vi "00_action_FISH02.vi"(11 "Line":string) -> (0 "Command Error":errorcluster, 1 "Execution Return":errorcluster, 2 "Return":string, 3 "full log":string)   [LabVIEW 2019]
uses:
  device/device_global.vi
  device/KQZ1-MP.llb/KQZ1.lvclass
  device/RHEODYNE7970_ADN.llb/RD7970ADN.lvclass
  device/VICI EMHCA.llb/VICI EMHCA_10PORTS.lvclass
  device/MSP1C2.llb/MSP1C2.lvclass
  device/CAVRO_XC.llb/XC3P.lvclass
  device/SC300.llb/SC300.lvclass
  device/SV_LG16ch.llb/SV_LG16ch.lvclass
  device/TETECH_TC720.llb/TC720.lvclass
panel:
  out "Boolean":bool
  out "#number":i32
  out "#class":string
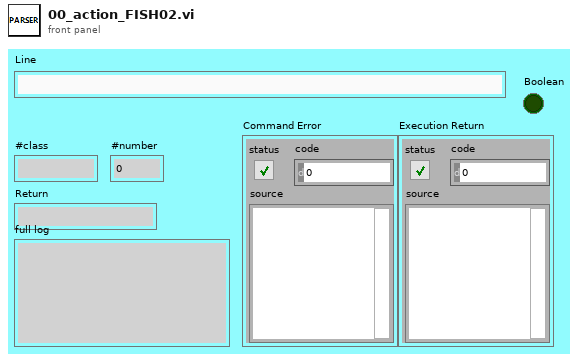
[diagram p1: front panel]
types:
  T1 = enum16{"open", "replace", "create", "open or create", "replace or create", "replace or create with confirmation"}
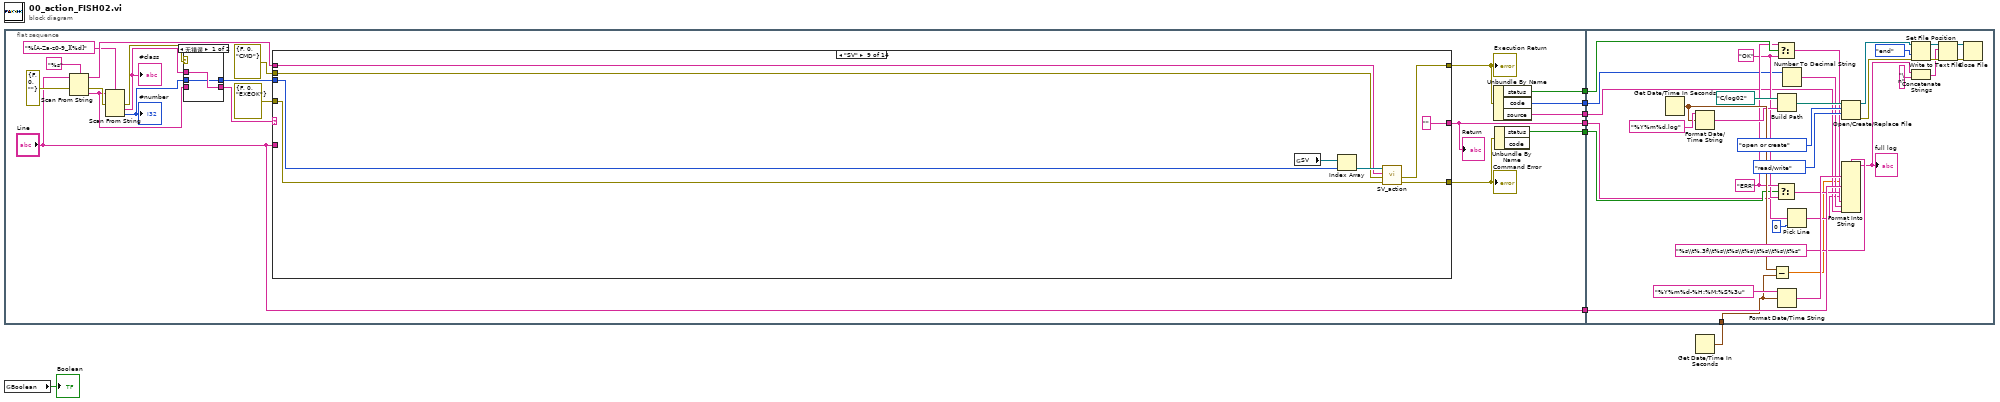
[diagram p0: block diagram]
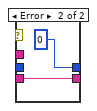
[diagram p2: hidden frame]
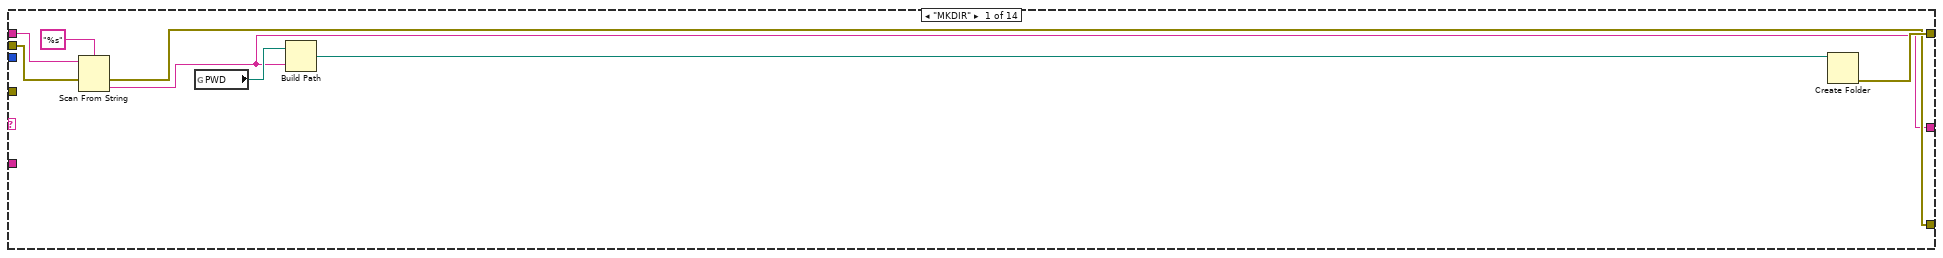
[diagram p3: hidden frame]
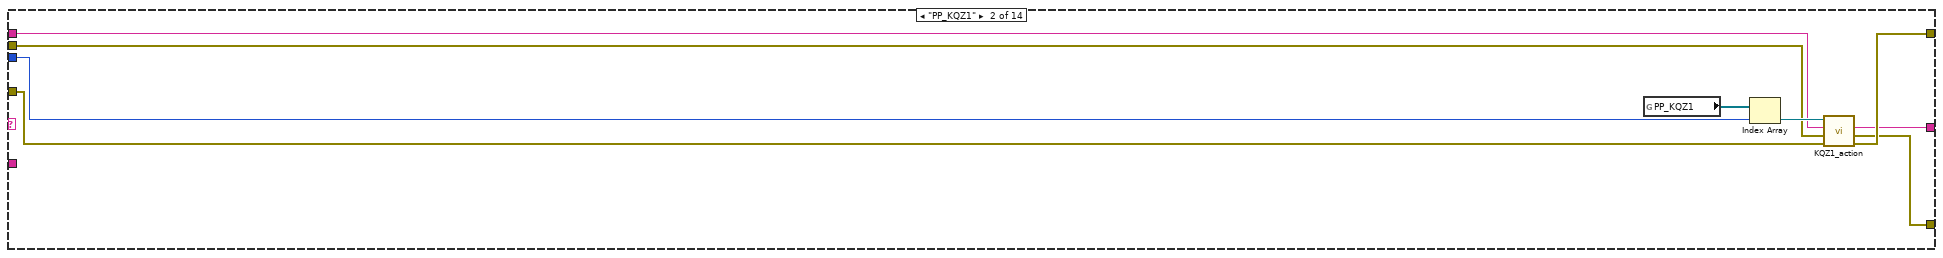
[diagram p4: hidden frame]
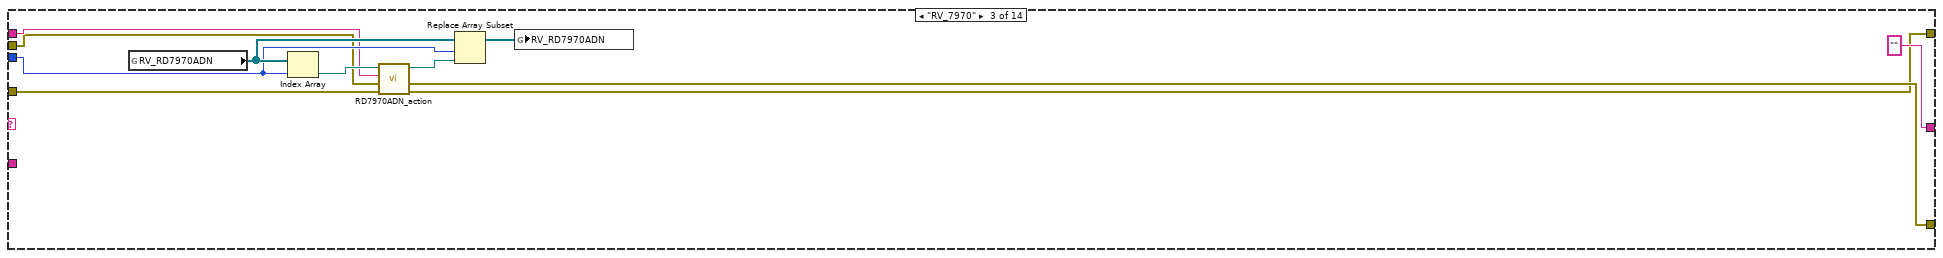
[diagram p5: hidden frame]
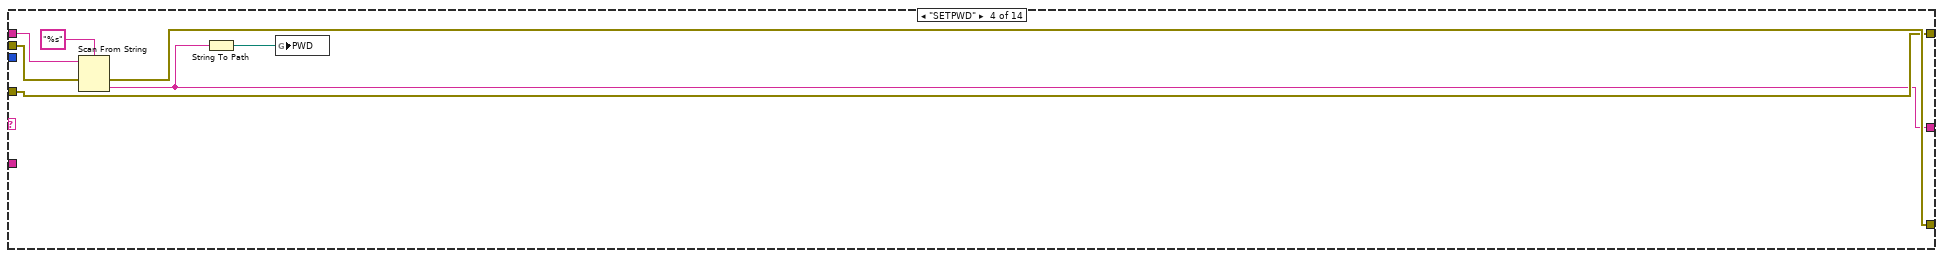
[diagram p6: hidden frame]
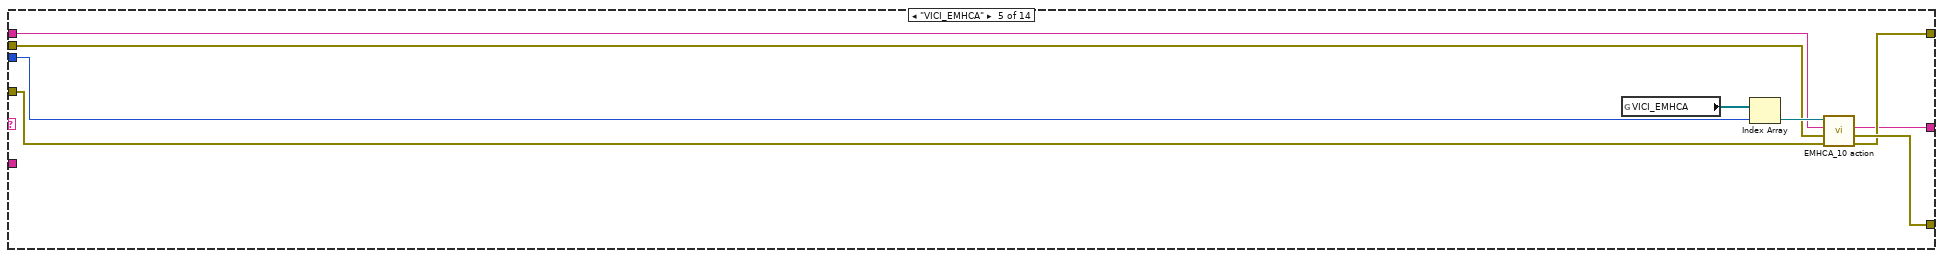
[diagram p7: hidden frame]
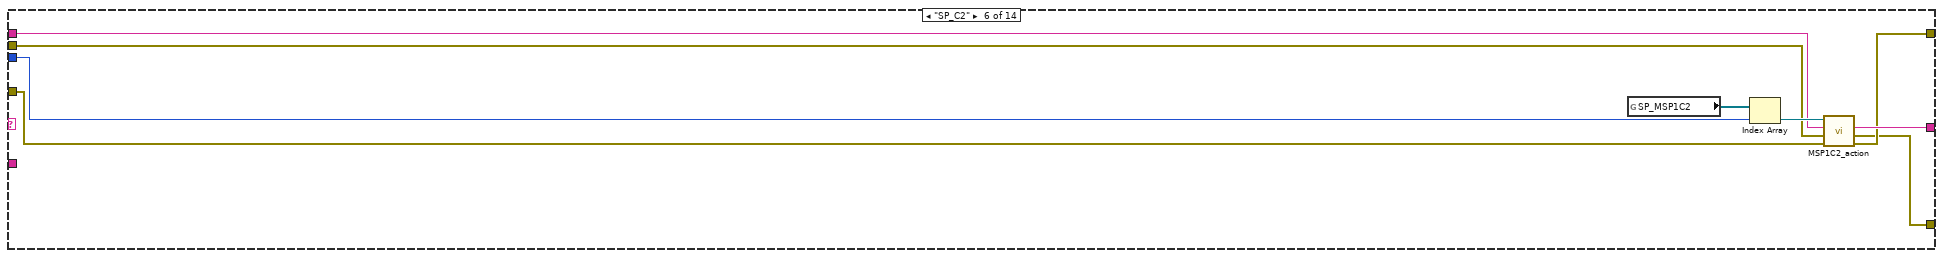
[diagram p8: hidden frame]
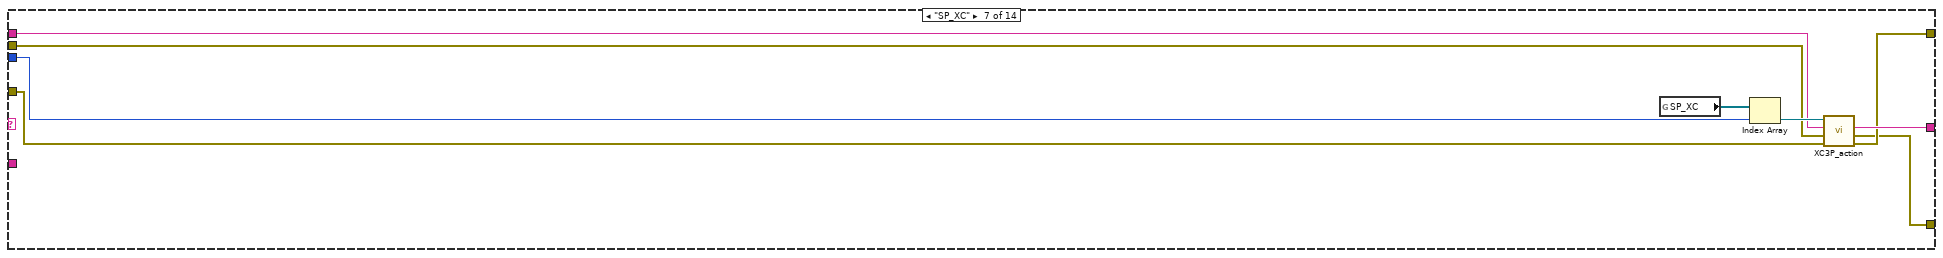
[diagram p9: hidden frame]
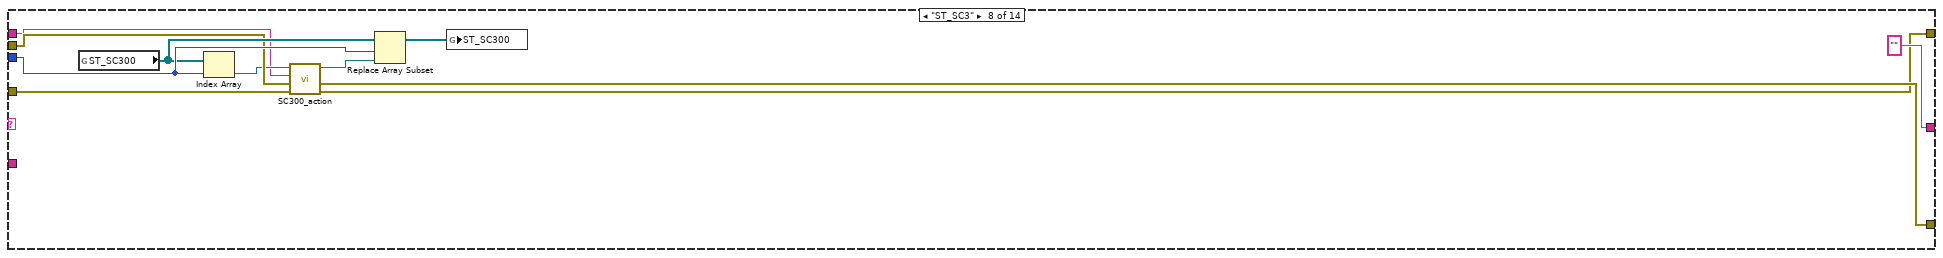
[diagram p10: hidden frame]
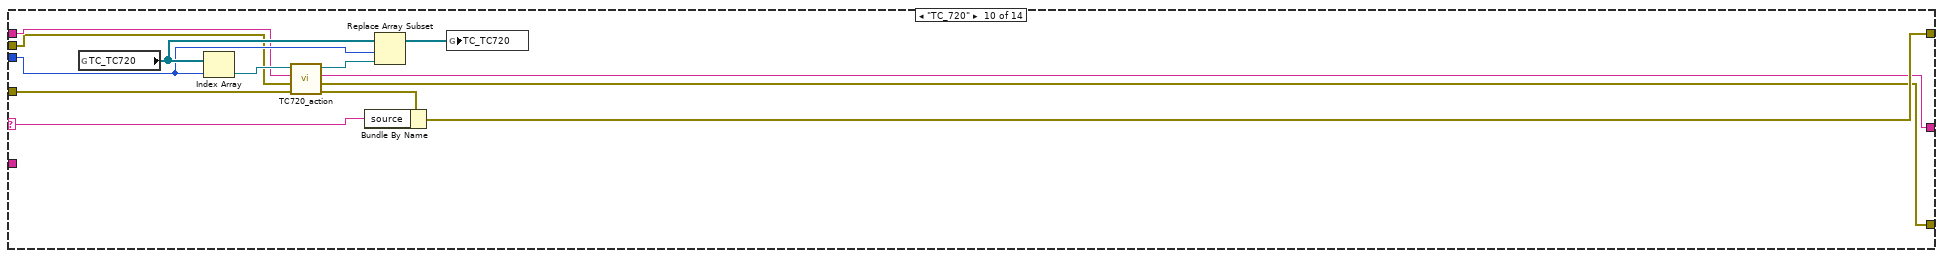
[diagram p11: hidden frame]
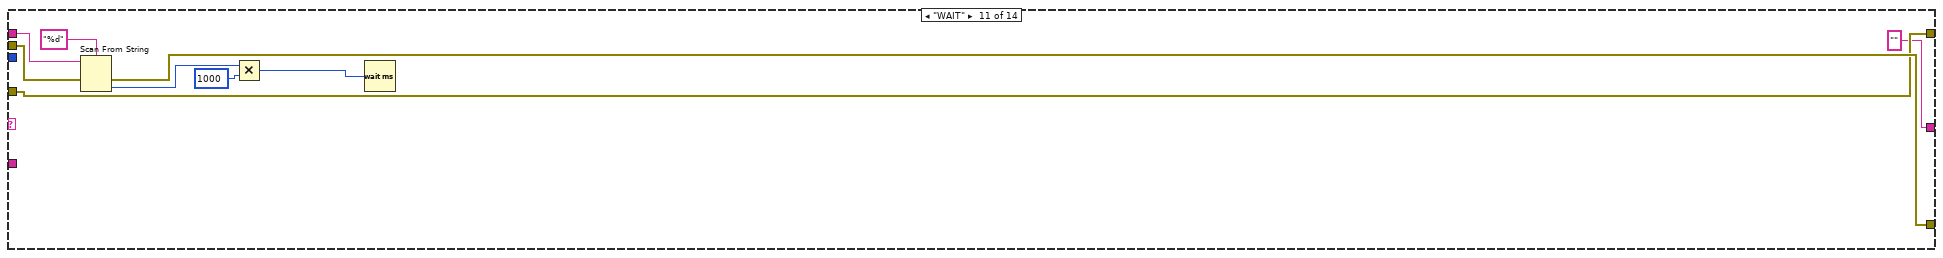
[diagram p12: hidden frame]
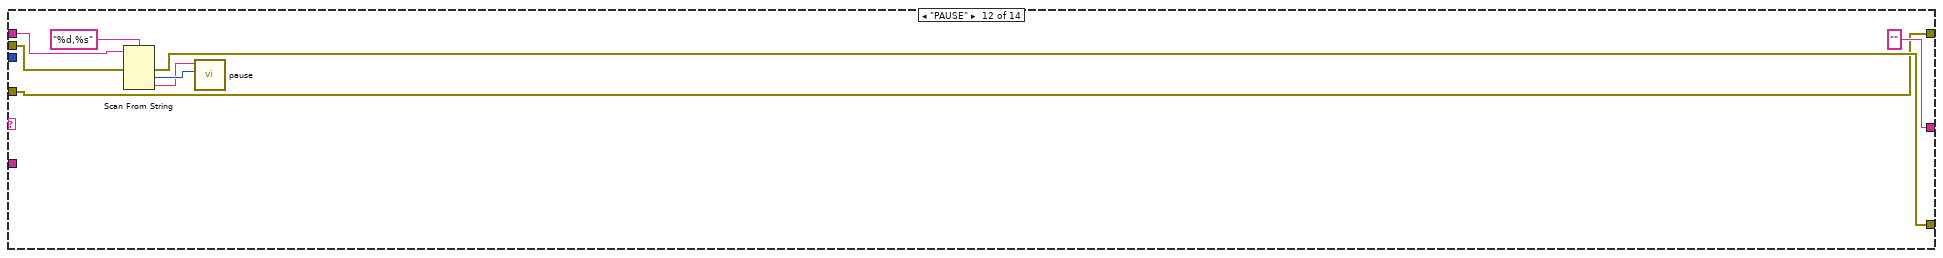
[diagram p13: hidden frame]
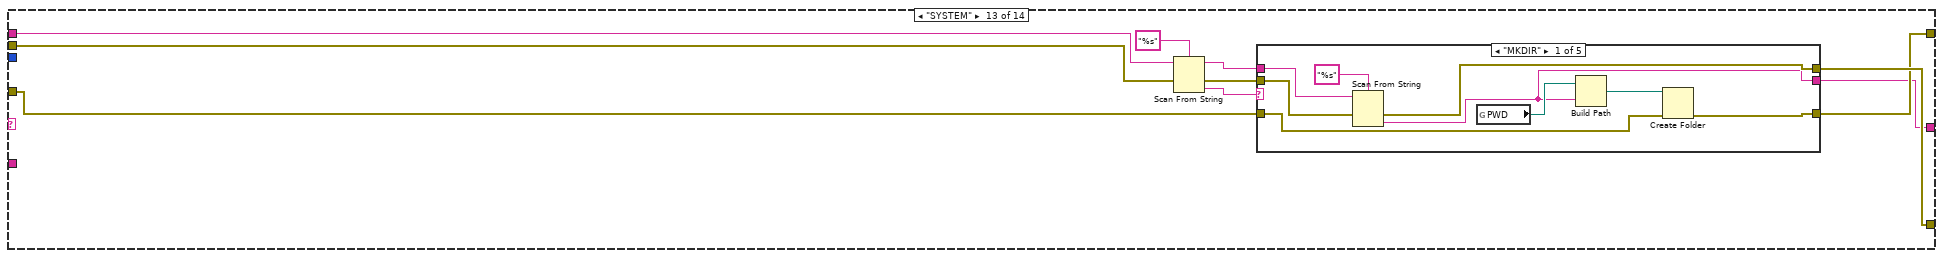
[diagram p14: hidden frame]
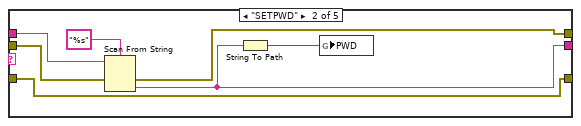
[diagram p15: hidden frame]
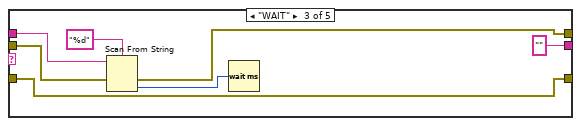
[diagram p16: hidden frame]
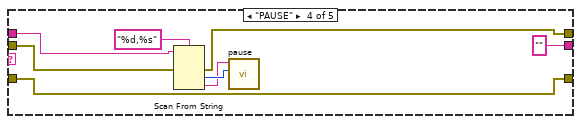
[diagram p17: hidden frame]
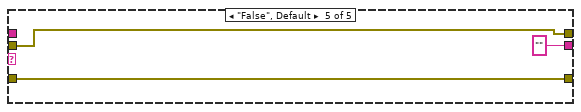
[diagram p18: hidden frame]
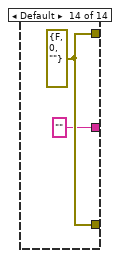
[diagram p19: hidden frame]
diagram:
  n1 = flat-sequence {
    tunnel: ["Line"] -> w7
    tunnel: [w15] -> w6
    tunnel: [w13] -> w5
    tunnel: [w11] -> w4
    tunnel: [w10] -> w2
    tunnel: [w9] -> w1
    tunnel: w8 -> [w223]
    tunnel: w7 -> [w226]
    tunnel: w6 -> [w194]
    tunnel: w5 -> [w200]
    tunnel: w4 -> [w204]
    tunnel: w2 -> [w197]
    tunnel: w1 -> [w198]
    frame #0 {
      n2 = Scan From String(format string="%s", input string="Line", error in=errorcluster {"status"=FALSE, "code"=0, "source"=""} ("error in (no error)")) -> (remaining string=w28:string, error out=w26:errorcluster, output 1=w21:string)  [unwired: 2 in, 1 out]
      n3 = Scan From String(format string="%[A-Za-z0-9_][%d]", input string=w21, error in=w26) -> (error out=w24:errorcluster, output 1=w23:string, output 2=w20:i32)  [unwired: 3 in, 2 out]
      "#class" <- w23
      "#number" <- w20
      n4 = case shown="无错误" w24 {
        tunnel: w23 -> [w31 _]
        tunnel: [w31 w33] -> w22
        tunnel: w21 -> [_ w33]
        tunnel: [w30 0 ("#number")] -> w19
        tunnel: w20 -> [w30 _]
        frame No Error {
        }
        frame Error {
        }
      }
      n5 = case shown="\"SV\"" w22 {
        selector: w22 -> [_ _ _ _ _ _ _ _ _ w125 _ _ _ _]
        tunnel: w28 -> [w40 w47 w54 w68 w74 w80 w89 w96 w107 w117 w133 w142 w150 _]
        tunnel: "Line" -> [_ _ _ _ _ _ _ _ _ _ _ _ _ _]
        tunnel: [w36 w44 w51 w63 w70 w83 w92 w100 w111 w126 w134 w138 w147 w191] -> w12
        tunnel: errorcluster {"status"=FALSE, "code"=0, "source"="EXEOK"} ("error in (no error)") -> [_ w45 w55 w63 w72 w78 w87 w98 w109 w118 w134 w138 w149 _]
        tunnel: [w35 w43 w52 w65 w71 w82 w91 w101 w112 w120 w135 w139 w148 w191] -> w14
        tunnel: errorcluster {"status"=FALSE, "code"=0, "source"="CMD"} ("error in (no error)") -> [w39 w46 w53 w64 w73 w79 w88 w99 w108 w116 w136 w144 w152 _]
        tunnel: w19 -> [_ w49 w59 _ w75 w85 w94 w106 w114 w124 _ _ _ _]
        tunnel: [w34 w42 "" ("read buffer") w62 w69 w84 w93 "" ("read buffer") "" ("read buffer") w122 "" ("read buffer") "" ("read buffer") w146 ""] -> w15
        frame "MKDIR" {
          n6 = Scan From String(format string="%s", input string=w40, error in=w39) -> (error out=w35:errorcluster, output 1=w34:string)  [unwired: 2 in, 2 out]
          n7 = global read "device_global.vi" "PWD"() -> (w38:path)
          n8 = Build Path(base path=w38, name or relative path=w34) -> (appended path=w37:path)
          n9 = Create Folder(path (use dialog)=w37) -> (error out=w36:errorcluster)  [unwired: 2 in, 2 out]
        }
        frame "PP_KQZ1" {
          n10 = global read "device_global.vi" "PP_KQZ1"() -> (w50:refnum<class "KQZ1.lvclass">[])
          n11 = Index Array(array=w50, index=w49) -> (element=w48:refnum<class "KQZ1.lvclass">)
          n12 = call-dynamic "KQZ1_action.vi"("error in (no error)"=w45, "error in (no error) 2"=w46, "input string"=w47, "KQZ1 in"=w48) -> ("error out"=w44:errorcluster, "error out 2"=w43:errorcluster, "read buffer"=w42:string)  [unwired: 4 in, 1 out]
        }
        frame "RV_7970" {
          n13 = global read "device_global.vi" "RV_RD7970ADN"() -> (w60:refnum<class "RD7970ADN.lvclass">[])
          n14 = Index Array(array=w60, index=w59) -> (element=w57:refnum<class "RD7970ADN.lvclass">)
          n15 = call-dynamic "RD7970ADN_action.vi"("error in (no error)"=w55, "error in 2"=w53, "input string"=w54, "RD7970ADN in"=w57) -> ("error out"=w51:errorcluster, "error out 2"=w52:errorcluster, "RD7970ADN out"=w56:refnum<class "RD7970ADN.lvclass">)  [unwired: 4 in, 1 out]
          n16 = Replace Array Subset(array=w60, new element=w56, index=w59) -> (w58:refnum<class "RD7970ADN.lvclass">[])
          n17 = global write "device_global.vi" "RV_RD7970ADN"(w58) -> ()
        }
        frame "SETPWD" {
          n18 = Scan From String(format string="%s", input string=w68, error in=w64) -> (error out=w65:errorcluster, output 1=w62:string)  [unwired: 2 in, 2 out]
          n19 = String To Path(string=w62) -> (path=w66:path)
          n20 = global write "device_global.vi" "PWD"(w66) -> ()
        }
        frame "VICI_EMHCA" {
          n21 = global read "device_global.vi" "VICI_EMHCA"() -> (w76:refnum<class "VICI EMHCA_10PORTS.lvclass">[])
          n22 = Index Array(array=w76, index=w75) -> (element=w77:refnum<class "VICI EMHCA_10PORTS.lvclass">)
          n23 = call-dynamic "EMHCA_10 action.vi"("error in (no error)"=w72, "error in (no error) 2"=w73, "input string"=w74, "VICI EMHCA_10PORTS in"=w77) -> ("error out"=w70:errorcluster, "error out 2"=w71:errorcluster, "output string"=w69:string)  [unwired: 4 in, 1 out]
        }
        frame "SP_C2" {
          n24 = global read "device_global.vi" "SP_MSP1C2"() -> (w86:refnum<class "MSP1C2.lvclass">[])
          n25 = Index Array(array=w86, index=w85) -> (element=w81:refnum<class "MSP1C2.lvclass">)
          n26 = call-dynamic "MSP1C2_action.vi"("error in (no error)"=w78, "error in (no error) 2"=w79, "input string"=w80, "MSP1C2 in"=w81) -> ("error out"=w83:errorcluster, "error out 2"=w82:errorcluster, "read buffer"=w84:string)  [unwired: 4 in, 1 out]
        }
        frame "SP_XC" {
          n27 = global read "device_global.vi" "SP_XC"() -> (w95:refnum<class "XC3P.lvclass">[])
          n28 = Index Array(array=w95, index=w94) -> (element=w90:refnum<class "XC3P.lvclass">)
          n29 = call-dynamic "XC3P_action.vi"("error in (no error)"=w87, "error in (no error) 2"=w88, "input string"=w89, "XC3P in"=w90) -> ("error out"=w92:errorcluster, "error out 2"=w91:errorcluster, "read buffer"=w93:string)  [unwired: 4 in, 1 out]
        }
        frame "ST_SC3" {
          n30 = global read "device_global.vi" "ST_SC300"() -> (w105:refnum<class "SC300.lvclass">[])
          n31 = Index Array(array=w105, index=w106) -> (element=w97:refnum<class "SC300.lvclass">)
          n32 = call-dynamic "SC300_action.vi"("error in (no error)"=w98, "error in (no error) 2"=w99, "input string"=w96, "SC300 in"=w97) -> ("error out"=w100:errorcluster, "error out 2"=w101:errorcluster, "SC300 out"=w102:refnum<class "SC300.lvclass">)  [unwired: 4 in, 1 out]
          n33 = Replace Array Subset(array=w105, new element=w102, index=w106) -> (w104:refnum<class "SC300.lvclass">[])
          n34 = global write "device_global.vi" "ST_SC300"(w104) -> ()
        }
        frame "SV" {
          n35 = global read "device_global.vi" "SV"() -> (w115:refnum<class "SV_LG16ch.lvclass">[])
          n36 = Index Array(array=w115, index=w114) -> (element=w110:refnum<class "SV_LG16ch.lvclass">)
          n37 = call-dynamic "SV_action.vi"("error in (no error)"=w109, "error in (no error) 2"=w108, "input string"=w107, "SV_LG16ch in"=w110) -> ("error out"=w112:errorcluster, "error out 2"=w111:errorcluster)  [unwired: 4 in, 2 out]
        }
        frame "TC_720" {
          n38 = global read "device_global.vi" "TC_TC720"() -> (w128:refnum<class "TC720.lvclass">[])
          n39 = Index Array(array=w128, index=w124) -> (element=w119:refnum<class "TC720.lvclass">)
          n40 = call-dynamic "TC720_action.vi"("error in (no error)"=w118, "error in (no error) 2"=w116, "input string"=w117, "TC720 in"=w119) -> ("error out"=w121:errorcluster, "error out 2"=w120:errorcluster, "output string"=w122:string, "TC720 out"=w123:refnum<class "TC720.lvclass">)  [unwired: 4 in]
          n41 = Bundle By Name(cluster=w121, "source"=w125) -> (w126:errorcluster)
          n42 = Replace Array Subset(array=w128, new element=w123, index=w124) -> (w127:refnum<class "TC720.lvclass">[])
          n43 = global write "device_global.vi" "TC_TC720"(w127) -> ()
        }
        frame "WAIT" {
          n44 = Scan From String(format string="%d", input string=w133, error in=w136) -> (error out=w135:errorcluster, output 1=w131:i32)  [unwired: 2 in, 2 out]
          n45 = Multiply(x=w131, y=1000) -> (x*y=w130:i32)
          n46 = Wait (ms)(milliseconds to wait=w130) -> ()  [unwired: 1 out]
        }
        frame "PAUSE" {
          n47 = Scan From String(format string="%d,%s", input string=w142, error in=w144) -> (error out=w139:errorcluster, output 1=w143:i32, output 2=w141:string)  [unwired: 3 in, 2 out]
          n48 = call "pause.vi"("Timeout(s)"=w143, "Message"=w141) -> ()  [unwired: 10 in]
        }
        frame "SYSTEM" {
          n49 = Scan From String(format string="%s", input string=w150, error in=w152) -> (remaining string=w153:string, error out=w151:errorcluster, output 1=w154:string)  [unwired: 2 in, 1 out]
          n50 = case shown="\"MKDIR\"" w154 {
            tunnel: w153 -> [w161 w168 w176 w183 _]
            tunnel: w151 -> [w160 w169 w175 w182 w187]
            tunnel: [w159 w167 w173 w179 w188] -> w147
            tunnel: [w158 w166 w174 w181 w187] -> w148
            tunnel: w149 -> [w157 w167 w173 w179 w188]
            tunnel: [w156 w165 "" "" ""] -> w146
            frame "MKDIR" {
              n51 = Scan From String(format string="%s", input string=w161, error in=w160) -> (error out=w158:errorcluster, output 1=w156:string)  [unwired: 2 in, 2 out]
              n52 = global read "device_global.vi" "PWD"() -> (w163:path)
              n53 = Build Path(base path=w163, name or relative path=w156) -> (appended path=w162:path)
              n54 = Create Folder(path (use dialog)=w162, error in=w157) -> (error out=w159:errorcluster)  [unwired: 1 in, 2 out]
            }
            frame "SETPWD" {
              n55 = Scan From String(format string="%s", input string=w168, error in=w169) -> (error out=w166:errorcluster, output 1=w165:string)  [unwired: 2 in, 2 out]
              n56 = String To Path(string=w165) -> (path=w170:path)
              n57 = global write "device_global.vi" "PWD"(w170) -> ()
            }
            frame "WAIT" {
              n58 = Scan From String(format string="%d", input string=w176, error in=w175) -> (error out=w174:errorcluster, output 1=w177:i32)  [unwired: 2 in, 2 out]
              n59 = Wait (ms)(milliseconds to wait=w177) -> ()  [unwired: 1 out]
            }
            frame "PAUSE" {
              n60 = Scan From String(format string="%d,%s", input string=w183, error in=w182) -> (error out=w181:errorcluster, output 1=w185:i32, output 2=w184:string)  [unwired: 3 in, 2 out]
              n61 = call "pause.vi"("Timeout(s)"=w185, "Message"=w184) -> ()  [unwired: 10 in]
            }
            frame "False", Default {
            }
          }
        }
        frame Default {
          w191 = errorcluster {"status"=FALSE, "code"=0, "source"=""} ("error IO")
        }
      }
      "Command Error" <- w14
      "Execution Return" <- w12
      "Return" <- w15
      n62 = Unbundle By Name(w12) -> ("status"=w11:bool, "code"=w10:i32, "source"=w9:string)
      n63 = Unbundle By Name(w14) -> ("status"=w13:bool)  [unwired: 1 out]
    }
    frame #1 {
      w201 = "OK" ("time format string (%c)")
      w202 = "ERR" ("time format string (%c)")
      n64 = Get Date/Time In Seconds() -> (seconds since 1Jan1904=w206:timestamp)
      n65 = Format Date/Time String(time format string (%c)="%Y%m%d.log", seconds (now)=w206) -> (date/time string=w205:string)  [unwired: 1 in]
      n66 = Subtract(x=w206, y=w223) -> (x-y=w192:dbl)
      n67 = Select(t=w202, s=w204, f=w201) -> (s? t:f=w203:string)
      n68 = Select(t=w202, s=w200, f=w201) -> (s? t:f=w199:string)
      n69 = Format Date/Time String(time format string (%c)="%Y%m%d-%H:%M:%S%3u", seconds (now)=w223) -> (date/time string=w225:string)  [unwired: 1 in]
      n70 = Build Path(base path=path "C:/log02" ("file path (use dialog)"), name or relative path=w205) -> (appended path=w208:path)
      n71 = Number To Decimal String(number=w197) -> (decimal integer string=w196:string)  [unwired: 1 in]
      n72 = Pick Line(multi-line string=w194, line index=0) -> (output string=w193:string)  [unwired: 1 in]
      n73 = Open/Create/Replace File(file path (use dialog)=w208, operation (0:open)=T1."open or create", access (0:read/write)=enum16{"read/write", "read-only", "write-only"}."read/write") -> (refnum out=w218:refnum<file>, error out=w216:errorcluster)  [unwired: 3 in, 1 out]
      n74 = Format Into String(format string="%s\\t%.3f\\t%s\\t%s\\t%s\\t%s\\t%s\\t%s", w225, w192, w226, w199, w193, w203, w196, w198) -> (resulting string=w214:string)  [unwired: 2 in, 1 out]
      "full log" <- w214
      n75 = Set File Position(refnum=w218, from (0:start)=enum16{"start", "end", "current"}."end", error in=w216) -> (refnum out=w217:refnum<file>, error out=w215:errorcluster)  [unwired: 1 in]
      n76 = Concatenate Strings(w214, "\n" ("string")) -> (w210:string)
      n77 = Write to Text File(file (use dialog)=w217, text=w210, error in=w215) -> (refnum out=w212:refnum<file>, error out=w211:errorcluster)  [unwired: 1 in, 1 out]
      n78 = Close File(refnum=w212, error in=w211) -> ()  [unwired: 2 out]
    }
  }
  n79 = global read "device_global.vi" "Boolean"() -> (→"Boolean":bool)
  n80 = Get Date/Time In Seconds() -> (seconds since 1Jan1904=w8:timestamp)
